vi "数据上传Z010.vi"(1 "数据数组":string[](array[string]), 2 "合格Z010":bool) -> ()   [LabVIEW 2013]
panel:
  out "error out 2":errorcluster
  out "Result 2":string caption="结果"
  out "Result":string
  in  "error in (no error)":errorcluster
  out "error out":errorcluster
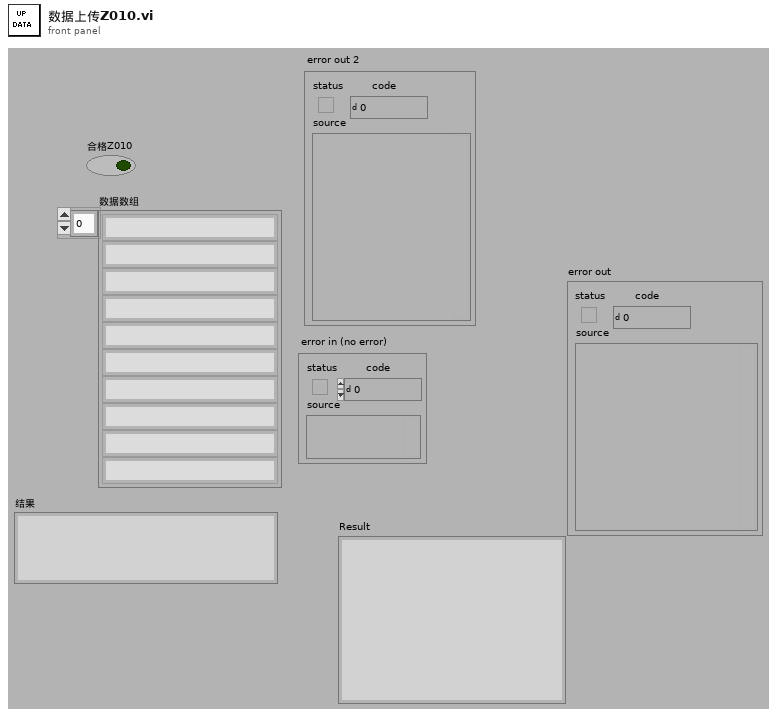
[diagram p1: front panel]
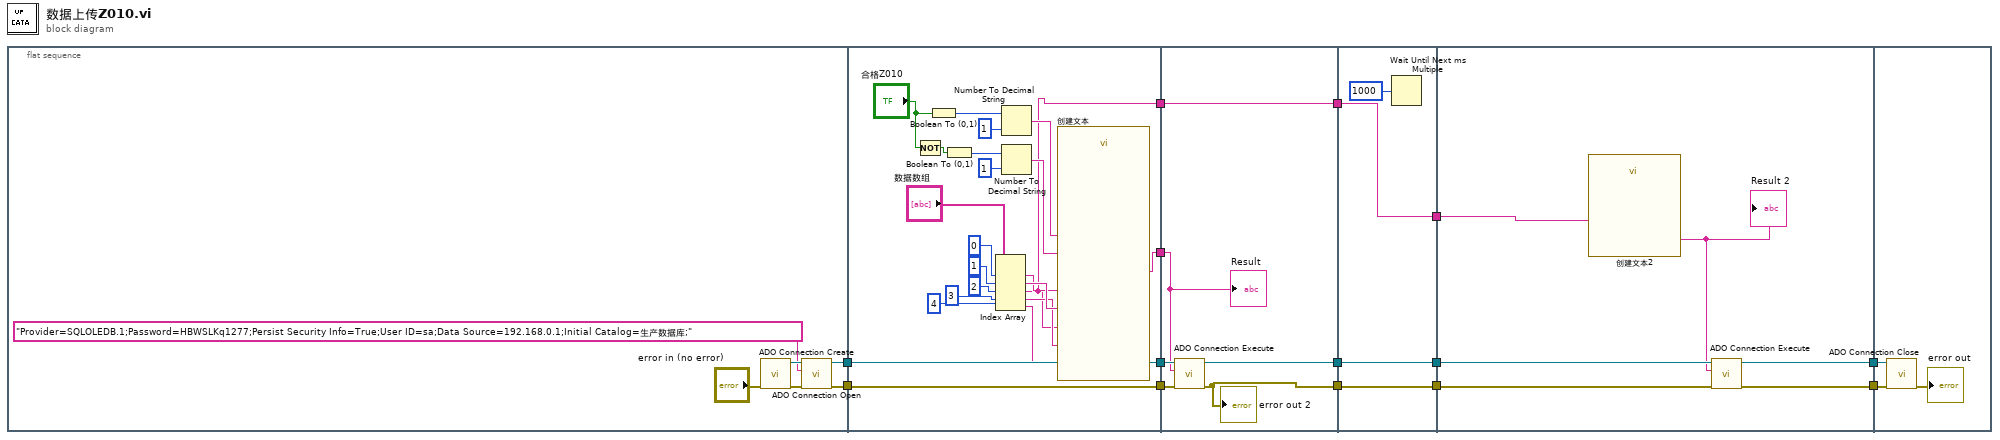
[diagram p0: block diagram]
diagram:
  n1 = flat-sequence {
    tunnel: [w16] -> w14
    tunnel: [w17] -> w13
    tunnel: w14 -> [w35]
    tunnel: w13 -> [w36]
    tunnel: [w36] -> w8
    tunnel: [w35] -> w6
    tunnel: [w26] -> w4
    tunnel: [w21] -> w1
    tunnel: w8 -> [w48]
    tunnel: [w44] -> w7
    tunnel: w6 -> [w46]
    tunnel: [w45] -> w5
    tunnel: w4 -> [w47]
    tunnel: [w43] -> w2
    tunnel: w1 -> [w43]
    tunnel: w7 -> [w52]
    tunnel: [w52] -> w12
    tunnel: w5 -> [w51]
    tunnel: [w51] -> w11
    tunnel: [w49] -> w3
    tunnel: w2 -> [w49]
    tunnel: w12 -> [w58]
    tunnel: w11 -> [w57]
    tunnel: [w55] -> w10
    tunnel: [w54] -> w9
    tunnel: w3 -> [w53]
    tunnel: w10 -> [w60]
    tunnel: w9 -> [w59]
    frame #0 {
      n2 = call "ADO Connection Create.vi"("error in (no error)"="error in (no error)") -> ("error out"=w19:errorcluster, "ADODB._Connection Out"=w18:refnum<k7>)  [unwired: 9 out]
      n3 = call "ADO Connection Open.vi"("error in (no error)"=w19, "ConnectionString"="Provider=SQLOLEDB.1;Password=HBWSLKq1277;Persist Security Info=True;User ID=sa;Data Source=192.168.0.1;Initial Catalog=生产数据库;" ("字符串 2"), "ADODB._Connection In"=w18) -> ("error out"=w16:errorcluster, "ADODB._Connection Out"=w17:refnum<k7>)  [unwired: 7 out]
    }
    frame #1 {
      n4 = Not(x="合格Z010") -> (.not. x?=w29:bool)
      n5 = Boolean To (0,1)(Boolean="合格Z010") -> (0, 1=w42:i16)
      n6 = Boolean To (0,1)(Boolean=w29) -> (0, 1=w28:i16)
      n7 = Index Array(array="数据数组", index #1=0 ("索引"), index #2=1 ("索引"), index #3=2 ("索引"), index #4=3 ("索引"), index #5=4 ("索引")) -> (element #1=w22:string, element #2=w25:string, element #3=w21:string, element #4=w24:string, element #5=w23:string)
      n8 = Number To Decimal String(number=w42, width (-)=i16 1 ("宽度(-)")) -> (decimal integer string=w37:string)
      n9 = Number To Decimal String(number=w28, width (-)=i16 1 ("宽度(-)")) -> (decimal integer string=w27:string)
      n10 = call "创建文本"("员工ID"=w25, "A实测监控点压力"=w24, "本序合格"=w37, "本序不合格"=w27, "结束时间"=w22, "壳体批次号"=w21, "B实测监控点压力"=w23) -> ("Result"=w26:string)  [unwired: 7 in, 1 out]
    }
    frame #2 {
      n11 = call "ADO Connection Execute.vi"("error in (no error)"=w46, "CommandText"=w47, "ADODB._Connection In"=w48) -> ("error out"=w45:errorcluster, "ADODB._Connection Out"=w44:refnum<k7>)  [unwired: 7 out]
      "error out 2" <- w45
      "Result" <- w47
    }
    frame #3 {
      n12 = Wait Until Next ms Multiple(millisecond multiple=u32 1000 ("毫秒倍数")) -> ()  [unwired: 1 out]
    }
    frame #4 {
      n13 = call "创建文本2"("壳体批次号"=w53) -> ("Result"=w56:string)  [unwired: 13 in, 1 out]
      "Result 2" <- w56
      n14 = call "ADO Connection Execute.vi"("error in (no error)"=w57, "CommandText"=w56, "ADODB._Connection In"=w58) -> ("error out"=w54:errorcluster, "ADODB._Connection Out"=w55:refnum<k7>)  [unwired: 7 out]
    }
    frame #5 {
      n15 = call "ADO Connection Close.vi"("error in (no error)"=w59, "ADODB._Connection In"=w60) -> ("error out"=→"error out":errorcluster)  [unwired: 9 out]
    }
  }
